vi "Load sxm File.vi"(8 "error in":errorcluster, 9 "Scan direction":bool=TRUE, 10 "Read channel":i8=-1 min=-1, 11 "Scan data file":path) -> (0 "error out":errorcluster, 1 "Data":sgl[][](array[numeric]) format="%#_5p", 2 "Channels info":T3, 3 "Scanfield":T2, 4 "Parameters":string[][](array[string]), 5 "Scan param":T1)   [LabVIEW 2017, in "Nanonis Prog Interface.lvlib"]
doc: "<B>Loads a Nanonis scan data (sxm) file.</B>\n\n<B>Scan data file</B>: path to the sxm file to load.\n<B>Read channel</B>: select which channel to read. If left unconnected, only the header information are read and no data are returned. To find out which channel to load you may run this function twice, using the <B>Channels config</B> output from the first run to determine the channel to load in the second run.\n<B>Scan direction</B>: defines whether to load the forward (True) or backward (False) data.\n\n\n<B>Scan param</B>: scan direction Up (True) or Down (False), scan speed in seconds per line, start time, and end time.\n<B>Channel data</B>: 2D-array containing the data of the specified channel and the given direction. The array element (0,0) corresponds to the top-left corner of the image.\n<B>Channels info</B>: list of channels available in the sxm file. Contains the channel name, calibration and offset. Use the channel indice in the <B>Read channel</B> input to load the data of that channel. Using calibration and offset you can calculate the voltage from the physical data.\n<B>Scanfield</B>: dimension of the scan field (center X & center Y, angle, width & height) and scan resolution (pixels & lines).\n<B>Parameters</B>: rest of header information.\n\n- Nanonis Programming Interface -"
uses:
  Nanonis Prog Interface.lvlib
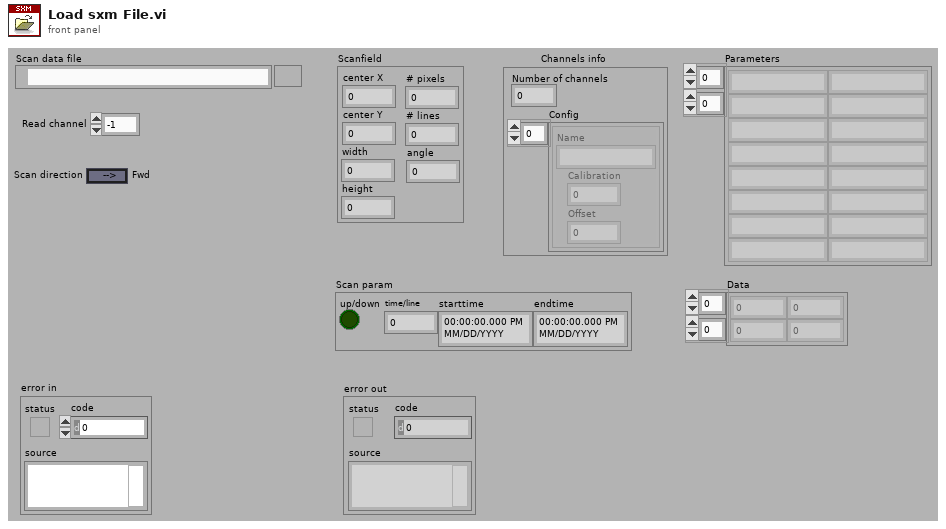
[diagram p1: front panel]
types:
  T1 = cluster{"up/down":bool, "time/line":sgl, "starttime":timestamp, "endtime":timestamp}
  T2 = cluster{"center X":sgl, "center Y":sgl, "angle":sgl, "width":sgl, "height":sgl, "# pixels":i32, "# lines":i32}
  T3 = cluster{"Number of channels":i8, "Config":cluster{"Name":string, "Calibration":sgl, "Offset":sgl}[]}
  T4 = enum16{"open", "replace", "create", "open or create", "replace or create", "replace or create with confirmation"}
  T5 = cluster{"Scanfield":cluster{"center X":sgl, "center Y":sgl, "width":sgl, "height":sgl, "angle":sgl}, "starttime":timestamp, "endtime":timestamp, "up/down":bool, "time/line":sgl, "selection":bool[], "# lines":i32, "# points":i32, "file":path, "channel config":cluster{"name":string, "calibration":sgl, "offset":sgl}[], "Parameters":string[][]}
  T6 = cluster{"name":string, "calibration":sgl, "offset":sgl}
  T7 = typedef "LVDateTimeRec.ctl" = cluster{"fractional second":dbl, "second":i32, "minute":i32, "hour":i32, "day of month":i32, "month":i32, "year":i32, "day of week":i32, "day of year":i32, "DST":i32}
  T8 = cluster{"name":string, "calibration":sgl, "offset":sgl}[]
  T9 = cluster{"center X":sgl, "center Y":sgl, "angle":sgl, "width":sgl, "height":sgl, "# points":i32, "# lines":i32}
  T10 = cluster{i32, "channel config":cluster{"name":string, "calibration":sgl, "offset":sgl}[]}
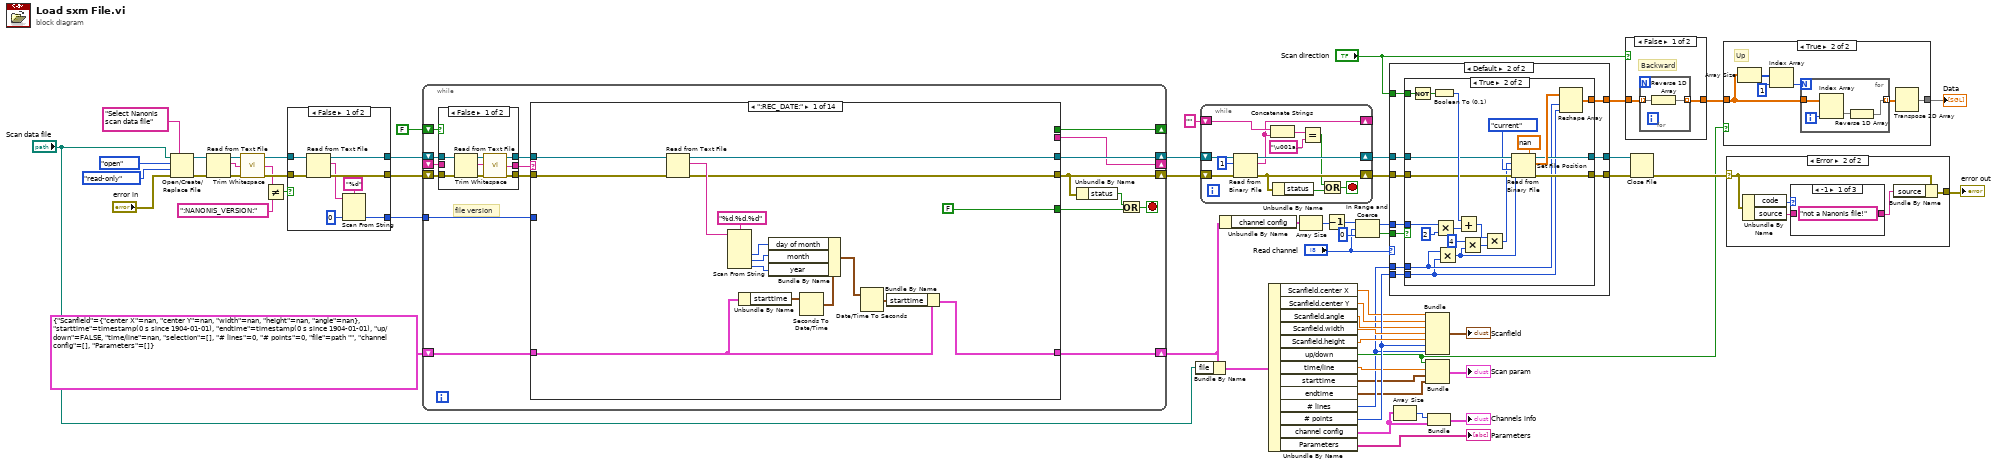
[diagram p0: block diagram]
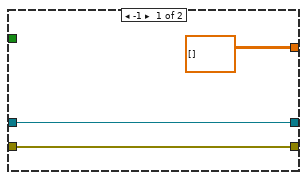
[diagram p4: hidden frame]
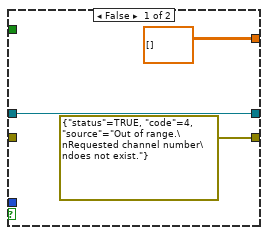
[diagram p5: hidden frame]
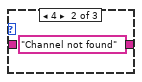
[diagram p7: hidden frame]
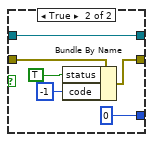
[diagram p9: hidden frame]
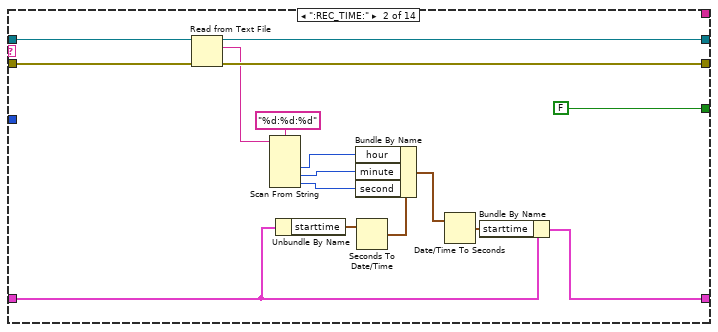
[diagram p11: hidden frame]
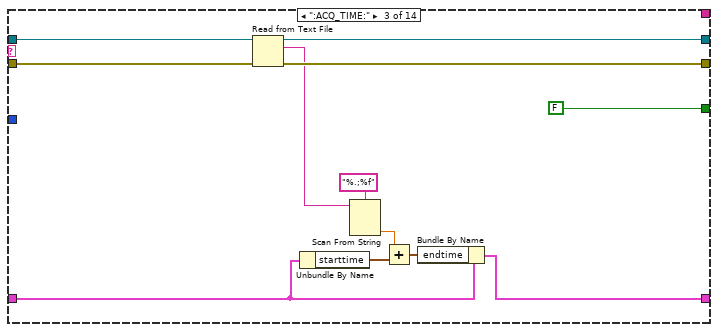
[diagram p12: hidden frame]
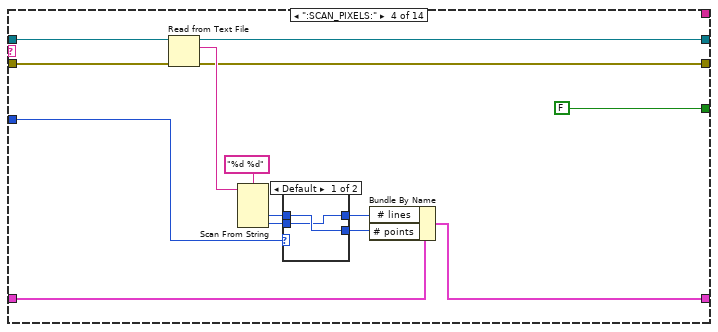
[diagram p13: hidden frame]
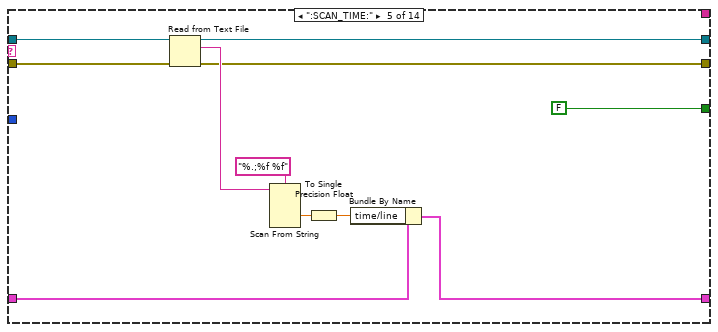
[diagram p15: hidden frame]
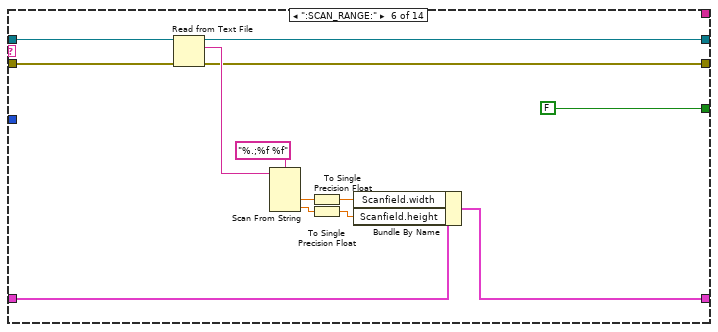
[diagram p16: hidden frame]
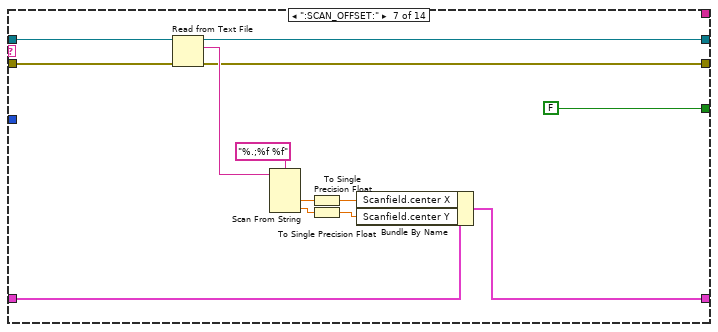
[diagram p17: hidden frame]
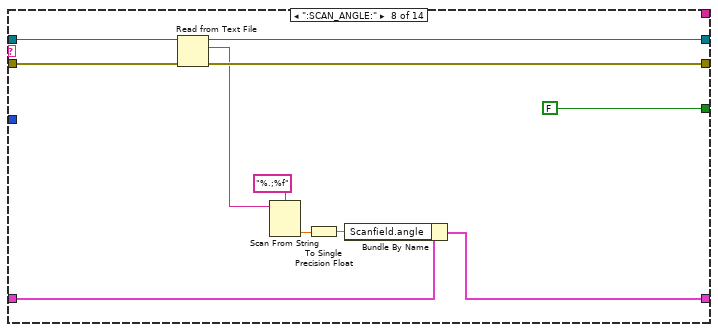
[diagram p18: hidden frame]
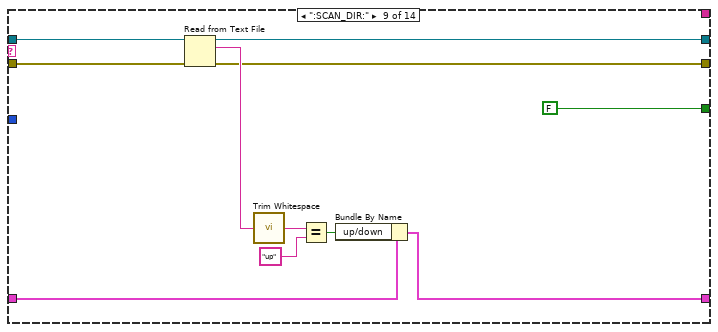
[diagram p19: hidden frame]
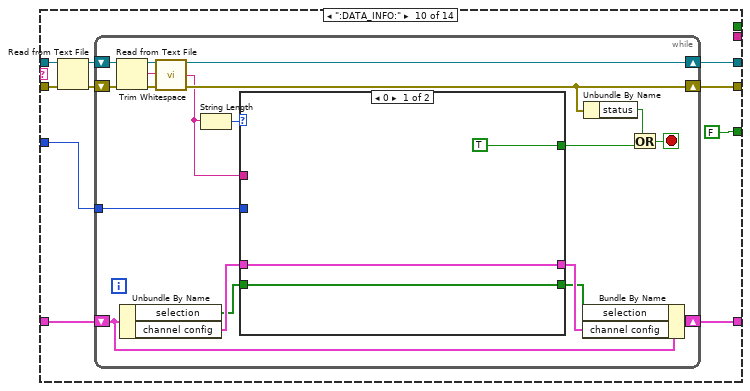
[diagram p20: hidden frame]
diagram:
  n1 = Open/Create/Replace File(file path (use dialog)="Scan data file", error in="error in", prompt="Select Nanonis scan data file", operation (0:open)=T4."open", access (0:read/write)=enum16{"read/write", "read-only", "write-only"}."read-only") -> (refnum out=w14:refnum<file>, error out=w15:errorcluster)  [unwired: 1 in, 1 out]
  n2 = Read from Text File(file (use dialog)=w14, error in=w15) -> (refnum out=w37:refnum<file>, text=w39:string, error out=w48:errorcluster)  [unwired: 2 in, 1 out]
  n3 = call <vilib>:"Trim Whitespace.vi"("string"=w39) -> ("trimmed string"=w38:string)  [unwired: 1 in]
  n4 = Not Equal?(x=w38, y=":NANONIS_VERSION:") -> (x != y?=w55:bool)
  n5 = case shown="False" w55 {
    tunnel: w48 -> [w58 w71]
    tunnel: [w65 w70] -> w47
    tunnel: w37 -> [w59 w68]
    tunnel: [w64 w68] -> w36
    tunnel: [w61 0 ("default value 1")] -> w35
    frame False {
      n6 = Read from Text File(file (use dialog)=w59, error in=w58) -> (refnum out=w64:refnum<file>, text=w62:string, error out=w65:errorcluster)  [unwired: 2 in, 1 out]
      n7 = Scan From String(format string="%d", input string=w62, default 1=0 ("default value 1")) -> (output 1=w61:i32)  [unwired: 2 in, 3 out]
    }
    frame True {
      n8 = Bundle By Name(cluster=w71, "status"=TRUE, "code"=-1) -> (w70:errorcluster)
    }
  }
  n9 = while {
    shift-right: [w87] -> w25
    shift-left: T5 {"Scanfield"={"center X"=nan, "center Y"=nan, "width"=nan, "height"=nan, "angle"=nan}, "starttime"=timestamp(0 s since 1904-01-01), "endtime"=timestamp(0 s since 1904-01-01), "up/down"=FALSE, "time/line"=nan, "selection"=[], "# lines"=0, "# points"=0, "file"=path "", "channel config"=[], "Parameters"=[]} ("Scan-Databuffer-attributes") -> [w88]
    shift-right: [w83] -> w52
    shift-left: w47 -> [w76]
    shift-right: [w79] -> w54
    shift-left: w36 -> [w77]
    tunnel: w35 -> [w78]
    shift-right: [w73] -> _
    shift-left: FALSE -> [w75]
    shift-right: [w72] -> _
    shift-left: _ -> [w74]
    stop <- w84 stop-if-true
    # "file version"
    n10 = case shown="False" w75 {
      tunnel: [w93 w96] -> w82
      tunnel: [w92 w95] -> w81
      tunnel: [w91 w97] -> w80
      tunnel: w77 -> [w90 w95]
      tunnel: w76 -> [w89 w96]
      tunnel: w74 -> [_ w97]
      frame False {
        n11 = Read from Text File(file (use dialog)=w90, error in=w89) -> (refnum out=w92:refnum<file>, text=w94:string, error out=w93:errorcluster)  [unwired: 2 in, 1 out]
        n12 = call <vilib>:"Trim Whitespace.vi"("string"=w94) -> ("trimmed string"=w91:string)  [unwired: 1 in]
      }
      frame True {
      }
    }
    n13 = case shown="\":REC_DATE:\"" w80 {
      selector: w80 -> [_ _ _ _ _ _ _ _ _ _ _ _ _ w347]
      tunnel: w81 -> [w101 w116 w131 w143 w161 w172 w185 w197 w209 w220 w311 w332 w344 w371]
      tunnel: [FALSE ("true") FALSE ("true") FALSE ("true") FALSE ("true") FALSE ("true") FALSE ("true") FALSE ("true") FALSE ("true") FALSE ("true") FALSE ("true") FALSE ("true") FALSE ("true") TRUE ("true") FALSE ("true")] -> w85
      tunnel: w88 -> [w112 w128 w141 w155 w170 w183 w196 w207 w218 w223 w303 w316 w345 w367]
      tunnel: [w111 w127 w140 w154 w169 w182 w195 w206 w217 w222 w301 w315 w345 w365] -> w87
      tunnel: [w104 w120 w133 w151 w165 w177 w190 w202 w212 w228 w313 w334 w344 w364] -> w79
      tunnel: w82 -> [w100 w117 w130 w142 w160 w171 w184 w198 w208 w219 w310 w331 w343 w370]
      tunnel: [w102 w119 w134 w149 w163 w175 w188 w201 w210 w224 w312 w333 w343 w363] -> w83
      tunnel: w78 -> [_ _ _ w144 _ _ _ _ _ w221 _ _ _ _]
      tunnel: [_ _ _ _ _ _ _ _ _ _ _ _ _ w362] -> w72
      tunnel: [_ _ _ _ _ _ _ _ _ _ _ _ _ w361] -> w73
      frame ":REC_DATE:" {
        n14 = Read from Text File(file (use dialog)=w101, error in=w100) -> (refnum out=w104:refnum<file>, text=w103:string, error out=w102:errorcluster)  [unwired: 2 in, 1 out]
        n15 = Scan From String(format string="%d.%d.%d", input string=w103) -> (output 1=w108:i32, output 2=w107:i32, output 3=w106:i32)  [unwired: 5 in, 3 out]
        n16 = Unbundle By Name(w112) -> ("starttime"=w99:timestamp)
        n17 = Seconds To Date/Time(time stamp (now)=w99) -> (date time rec=w113:T7)  [unwired: 1 in]
        n18 = Bundle By Name(cluster=w113, "day of month"=w108, "month"=w107, "year"=w106) -> (w98:T7)
        n19 = Date/Time To Seconds(2:w98) -> (0:w110:timestamp)  [unwired: 1 in]
        n20 = Bundle By Name(cluster=w112, "starttime"=w110) -> (w111:T5)
      }
      frame ":REC_TIME:" {
        n21 = Read from Text File(file (use dialog)=w116, error in=w117) -> (refnum out=w120:refnum<file>, text=w118:string, error out=w119:errorcluster)  [unwired: 2 in, 1 out]
        n22 = Scan From String(format string="%d:%d:%d", input string=w118) -> (output 1=w124:i32, output 2=w123:i32, output 3=w122:i32)  [unwired: 5 in, 3 out]
        n23 = Unbundle By Name(w128) -> ("starttime"=w115:timestamp)
        n24 = Seconds To Date/Time(time stamp (now)=w115) -> (date time rec=w129:T7)  [unwired: 1 in]
        n25 = Bundle By Name(cluster=w129, "hour"=w124, "minute"=w123, "second"=w122) -> (w114:T7)
        n26 = Date/Time To Seconds(2:w114) -> (0:w126:timestamp)  [unwired: 1 in]
        n27 = Bundle By Name(cluster=w128, "starttime"=w126) -> (w127:T5)
      }
      frame ":ACQ_TIME:" {
        n28 = Read from Text File(file (use dialog)=w131, error in=w130) -> (refnum out=w133:refnum<file>, text=w132:string, error out=w134:errorcluster)  [unwired: 2 in, 1 out]
        n29 = Unbundle By Name(w141) -> ("starttime"=w137:timestamp)
        n30 = Scan From String(format string="%.;%f", input string=w132) -> (output 1=w135:dbl)  [unwired: 3 in, 3 out]
        n31 = Add(x=w135, y=w137) -> (x+y=w136:timestamp)
        n32 = Bundle By Name(cluster=w141, "endtime"=w136) -> (w140:T5)
      }
      frame ":SCAN_PIXELS:" {
        n33 = Read from Text File(file (use dialog)=w143, error in=w142) -> (refnum out=w151:refnum<file>, text=w150:string, error out=w149:errorcluster)  [unwired: 2 in, 1 out]
        n34 = Scan From String(format string="%d %d", input string=w150) -> (output 1=w148:i32, output 2=w147:i32)  [unwired: 4 in, 3 out]
        n35 = case shown="Default" w144 {
          tunnel: w148 -> [w157 w159]
          tunnel: w147 -> [w156 w158]
          tunnel: [w156 w159] -> w146
          tunnel: [w157 w158] -> w145
          frame Default {
          }
          frame 0, 1 {
          }
        }
        n36 = Bundle By Name(cluster=w155, "# lines"=w146, "# points"=w145) -> (w154:T5)
      }
      frame ":SCAN_TIME:" {
        n37 = Read from Text File(file (use dialog)=w161, error in=w160) -> (refnum out=w165:refnum<file>, text=w164:string, error out=w163:errorcluster)  [unwired: 2 in, 1 out]
        n38 = Scan From String(format string="%.;%f %f", input string=w164) -> (output 1=w167:dbl)  [unwired: 5 in, 3 out]
        n39 = To Single Precision Float(number=w167) -> (single precision float=w162:sgl)
        n40 = Bundle By Name(cluster=w170, "time/line"=w162) -> (w169:T5)
      }
      frame ":SCAN_RANGE:" {
        n41 = Read from Text File(file (use dialog)=w172, error in=w171) -> (refnum out=w177:refnum<file>, text=w176:string, error out=w175:errorcluster)  [unwired: 2 in, 1 out]
        n42 = Scan From String(format string="%.;%f %f", input string=w176) -> (output 1=w180:dbl, output 2=w179:dbl)  [unwired: 4 in, 3 out]
        n43 = To Single Precision Float(number=w180) -> (single precision float=w174:sgl)
        n44 = To Single Precision Float(number=w179) -> (single precision float=w173:sgl)
        n45 = Bundle By Name(cluster=w183, "Scanfield.width"=w174, "Scanfield.height"=w173) -> (w182:T5)
      }
      frame ":SCAN_OFFSET:" {
        n46 = Read from Text File(file (use dialog)=w185, error in=w184) -> (refnum out=w190:refnum<file>, text=w189:string, error out=w188:errorcluster)  [unwired: 2 in, 1 out]
        n47 = Scan From String(format string="%.;%f %f", input string=w189) -> (output 1=w193:dbl, output 2=w192:dbl)  [unwired: 4 in, 3 out]
        n48 = To Single Precision Float(number=w193) -> (single precision float=w187:sgl)
        n49 = To Single Precision Float(number=w192) -> (single precision float=w186:sgl)
        n50 = Bundle By Name(cluster=w196, "Scanfield.center X"=w187, "Scanfield.center Y"=w186) -> (w195:T5)
      }
      frame ":SCAN_ANGLE:" {
        n51 = Read from Text File(file (use dialog)=w197, error in=w198) -> (refnum out=w202:refnum<file>, text=w200:string, error out=w201:errorcluster)  [unwired: 2 in, 1 out]
        n52 = Scan From String(format string="%.;%f", input string=w200) -> (output 1=w204:dbl)  [unwired: 3 in, 3 out]
        n53 = To Single Precision Float(number=w204) -> (single precision float=w199:sgl)
        n54 = Bundle By Name(cluster=w207, "Scanfield.angle"=w199) -> (w206:T5)
      }
      frame ":SCAN_DIR:" {
        n55 = Read from Text File(file (use dialog)=w209, error in=w208) -> (refnum out=w212:refnum<file>, text=w211:string, error out=w210:errorcluster)  [unwired: 2 in, 1 out]
        n56 = call <vilib>:"Trim Whitespace.vi"("string"=w211) -> ("trimmed string"=w215:string)  [unwired: 1 in]
        n57 = Equal?(x=w215, y="up") -> (x = y?=w213:bool)
        n58 = Bundle By Name(cluster=w218, "up/down"=w213) -> (w217:T5)
      }
      frame ":DATA_INFO:" {
        n59 = Read from Text File(file (use dialog)=w220, error in=w219) -> (refnum out=w226:refnum<file>, error out=w225:errorcluster)  [unwired: 2 in, 2 out]
        n60 = while {
          shift-right: [w235] -> w222
          shift-left: w223 -> [w236]
          shift-right: [w242] -> w224
          shift-left: w225 -> [w229]
          shift-right: [w244] -> w228
          shift-left: w226 -> [w230]
          tunnel: w221 -> [w231]
          stop <- w239 stop-if-true
          n61 = Read from Text File(file (use dialog)=w230, error in=w229) -> (refnum out=w244:refnum<file>, text=w243:string, error out=w242:errorcluster)  [unwired: 2 in, 1 out]
          n62 = Unbundle By Name(w236) -> ("selection"=w234:bool[], "channel config"=w238:T8)
          n63 = call <vilib>:"Trim Whitespace.vi"("string"=w243) -> ("trimmed string"=w232:string)  [unwired: 1 in]
          n64 = String Length(string=w232) -> (length=w245:i32)
          n65 = case shown="0" w245 {
            tunnel: w238 -> [w248 w255]
            tunnel: [w248 w254] -> w237
            tunnel: [TRUE w253] -> w240
            tunnel: w234 -> [w246 w252]
            tunnel: [w246 w251] -> w233
            tunnel: w232 -> [_ w250]
            tunnel: w231 -> [_ w249]
            frame 0 {
            }
            frame Default {
              n66 = case shown="Default" w249 {
                tunnel: w255 -> [w274 w294]
                tunnel: [w272 w292] -> w254
                tunnel: [FALSE FALSE] -> w253
                tunnel: w252 -> [w268 w288]
                tunnel: [w266 w286] -> w251
                tunnel: w250 -> [w256 w277]
                frame 0, 1 {
                  w262 = "%.; %d%s%s%s%e%e"  # Read strings (no whitespace allowed)
                  n67 = Scan From String(format string=w262, input string=w256) -> (output 1=w261:i32, output 2=w260:string, output 3=w259:string, output 5=w258:dbl, output 6=w257:dbl)  [unwired: 9 in, 3 out]
                  n68 = Replace Array Subset(array=w268, new element=TRUE ("new element/subarray"), index=w261) -> (w266:bool[])
                  n69 = Search and Replace String(replace all?=TRUE ("replace all? (F)"), input string=w260, search string="_", replace string=" " ("replace string (\"\")")) -> (result string=w264:string)  [unwired: 4 in, 3 out]
                  n70 = call <userlib>:"Append Unit to Signal Name.vi"("Unit"=w259, "Name"=w264) -> ("Name with unit"=w263:string)  [unwired: 5 in]
                  n71 = Bundle By Name(cluster=T6 {"name"="", "calibration"=0.0, "offset"=0.0} ("channel config"), "name"=w263, "calibration"=w258, "offset"=w257) -> (w273:T6)
                  n72 = Build Array (concatenate)(w274, w273) -> (w272:T8)
                }
                frame Default {
                  w276 = "%.;%d\t%[^\t]\t%[^\t]\t%s\t%e\t%e"  # Read tab-separated strings (spaces allowed)
                  n73 = Scan From String(format string=w276, input string=w277) -> (output 1=w282:i32, output 2=w281:string, output 3=w280:string, output 5=w279:dbl, output 6=w278:dbl)  [unwired: 9 in, 3 out]
                  n74 = Replace Array Subset(array=w288, new element=TRUE ("new element/subarray"), index=w282) -> (w286:bool[])
                  n75 = Search and Replace String(replace all?=TRUE ("replace all? (F)"), input string=w281, search string="_", replace string=" " ("replace string (\"\")")) -> (result string=w284:string)  [unwired: 4 in, 3 out]
                  n76 = call <userlib>:"Append Unit to Signal Name.vi"("Unit"=w280, "Name"=w284) -> ("Name with unit"=w283:string)  [unwired: 5 in]
                  n77 = Bundle By Name(cluster=T6 {"name"="", "calibration"=0.0, "offset"=0.0} ("channel config"), "name"=w283, "calibration"=w279, "offset"=w278) -> (w293:T6)
                  n78 = Build Array (concatenate)(w294, w293) -> (w292:T8)
                }
              }
            }
          }
          n79 = Bundle By Name(cluster=w236, "selection"=w233, "channel config"=w237) -> (w235:T5)
          n80 = Unbundle By Name(w242) -> ("status"=w241:bool)
          n81 = Or(x=w241, y=w240) -> (x .or. y?=w239:bool)
        }
      }
      frame ":BIAS:" {
        n82 = Read from Text File(file (use dialog)=w311, error in=w310) -> (refnum out=w313:refnum<file>, text=w297:string, error out=w312:errorcluster)  [unwired: 2 in, 1 out]
        n83 = call <vilib>:"Trim Whitespace.vi"("string"=w297) -> ("trimmed string"=w296:string)  [unwired: 1 in]
        n84 = Scan From String(format string="%.;%f", input string=w297) -> (error out=w300:errorcluster, output 1=w307:dbl)  [unwired: 3 in, 2 out]
        n85 = Format Value(format string="%#_6p", value (0)=w307) -> (output string=w299:string)  [unwired: 1 in]
        n86 = Unbundle By Name(w303) -> ("Parameters"=w309:string[][])
        n87 = Select(t=w296, s=w300, f=w299) -> (s? t:f=w298:string)
        n88 = Build Array("Bias (V)" ("element"), w298) -> (w304:string[])
        n89 = Build Array (concatenate)(w309, w304) -> (w302:string[][])
        n90 = Bundle By Name(cluster=w303, "Parameters"=w302) -> (w301:T5)
      }
      frame ":Z-CONTROLLER:" {
        w322 = string[] []
        w323 = "%s" ("format string")
        w324 = "\t"
        n91 = Read from Text File(file (use dialog)=w332, error in=w331) -> (refnum out=w330:refnum<file>, text=w328:string, error out=w329:errorcluster)  [unwired: 2 in, 1 out]
        n92 = call <vilib>:"Trim Whitespace.vi"("string"=w328) -> ("trimmed string"=w326:string)  [unwired: 1 in]
        n93 = Spreadsheet String To Array(delimiter (Tab)=w324, format string=w323, spreadsheet string=w326, array type (2D Dbl)=w322) -> (array=w320:string[])
        n94 = Read from Text File(file (use dialog)=w330, error in=w329) -> (refnum out=w334:refnum<file>, text=w327:string, error out=w333:errorcluster)  [unwired: 2 in, 1 out]
        n95 = call <vilib>:"Trim Whitespace.vi"("string"=w327) -> ("trimmed string"=w325:string)  [unwired: 1 in]
        n96 = Spreadsheet String To Array(delimiter (Tab)=w324, format string=w323, spreadsheet string=w325, array type (2D Dbl)=w322) -> (array=w319:string[])
        n97 = Unbundle By Name(w316) -> ("Parameters"=w318:string[][])
        n98 = for {
          tunnel: "Z-Ctrl: " ("string") -> [w342]
          tunnel: w320 -> [w341] mode=indexing
          tunnel: w319 -> [w339] mode=indexing
          shift-right: [w338] -> w317
          shift-left: w318 -> [w337]
          n99 = Concatenate Strings(w342, w341) -> (w340:string)
          n100 = Build Array(w340, w339) -> (w336:string[])
          n101 = Build Array (concatenate)(w337, w336) -> (w338:string[][])
        }
        n102 = Bundle By Name(cluster=w316, "Parameters"=w317) -> (w315:T5)
      }
      frame ":SCANIT_END:" {
      }
      frame Default {
        n103 = while {
          tunnel: w371 -> [w385]
          tunnel: w370 -> [w384]
          tunnel: [w383] -> w364
          tunnel: [w380] -> w363
          tunnel: [w373] -> w362
          tunnel: [w377] -> w361
          shift-right: [w374] -> w359
          shift-left: "" -> [w375]
          stop <- w379 stop-if-true
          n104 = Read from Text File(file (use dialog)=w385, error in=w384) -> (refnum out=w383:refnum<file>, text=w376:string, error out=w380:errorcluster)  [unwired: 2 in, 1 out]
          n105 = Match Pattern(string=w376, regular expression="^:.*:") -> (match substring=w373:string, offset past match=w381:i32)  [unwired: 1 in, 2 out]
          n106 = Unbundle By Name(w380) -> ("status"=w378:bool)
          n107 = Greater Or Equal To 0?(x=w381) -> (x >= 0?=w377:bool)
          n108 = Or(x=w377, y=w378) -> (x .or. y?=w379:bool)
          n109 = case shown="False" w377 {
            tunnel: w376 -> [w388 _]
            tunnel: w375 -> [w387 w389]
            tunnel: [w386 w389] -> w374
            frame False {
              n110 = Concatenate Strings(w387, w388) -> (w386:string)
            }
            frame True {
            }
          }
        }
        n111 = String Length(string=w347) -> (length=w353:i32)
        n112 = Subtract(x=w353, y=2) -> (x-y=w351:i32)
        n113 = String Subset(string=w347, offset (0)=1, length (rest)=w351) -> (substring=w350:string)
        n114 = Match Pattern(string=w347, regular expression=":.*:") -> (offset past match=w356:i32)  [unwired: 1 in, 3 out]
        n115 = Empty String/Path?(string/path=w347) -> (empty?=w369:bool)
        n116 = Less Than 0?(x=w356) -> (x < 0?=w355:bool)
        n117 = Unbundle By Name(w367) -> ("Parameters"=w368:string[][])
        n118 = call <vilib>:"Trim Whitespace.vi"("string"=w359) -> ("trimmed string"=w349:string)  [unwired: 1 in]
        n119 = Select(t=w347, s=w355, f=w350) -> (s? t:f=w348:string)
        n120 = Build Array(w348, w349) -> (w358:string[])
        n121 = case shown="False" w369 {
          tunnel: w368 -> [w391 w393]
          tunnel: [w392 w393] -> w366
          tunnel: w358 -> [w390 _]
          frame False {
            n122 = Build Array (concatenate)(w391, w390) -> (w392:string[][])
          }
          frame True {
          }
        }
        n123 = Bundle By Name(cluster=w367, "Parameters"=w366) -> (w365:T5)
      }
    }
    n124 = Unbundle By Name(w83) -> ("status"=w86:bool)
    n125 = Or(x=w86, y=w85) -> (x .or. y?=w84:bool)
  }
  n126 = Bundle By Name(cluster=w25, "file"="Scan data file") -> (w34:T5)
  n127 = while {
    shift-right: [w400] -> _
    shift-left: "" -> [w405]
    shift-right: [w401] -> w50
    shift-left: w52 -> [w395]
    shift-right: [w403] -> w51
    shift-left: w54 -> [w396]
    stop <- w397 stop-if-true
    n128 = Read from Binary File(8:w395, 10:1 ("count"), 11:w396) -> (0:w401:errorcluster, 2:w400:string, 3:w403:refnum<file>)  [unwired: 3 in, 1 out]
    n129 = Concatenate Strings(w405, w400) -> (w404:string)
    n130 = Unbundle By Name(w401) -> ("status"=w399:bool)
    n131 = Equal?(x=w404, y="\u001a\u0004") -> (x = y?=w398:bool)
    n132 = Or(x=w398, y=w399) -> (x .or. y?=w397:bool)
  }
  n133 = Unbundle By Name(w25) -> ("channel config"=w44:T8)
  n134 = Unbundle By Name(w34) -> ("Scanfield.center X"=w12:sgl, "Scanfield.center Y"=w11:sgl, "Scanfield.angle"=w10:sgl, "Scanfield.width"=w30:sgl, "Scanfield.height"=w29:sgl, "up/down"=w21:bool, "time/line"=w27:sgl, "starttime"=w3:timestamp, "endtime"=w2:timestamp, "# lines"=w4:i32, "# points"=w28:i32, "channel config"=w13:T8, "Parameters"=→"Parameters":string[][])
  n135 = Array Size(array=w44) -> (size(s)=w43:i32)
  n136 = Decrement(x=w43) -> (x-1=w42:i32)
  n137 = In Range and Coerce(upper limit=w42, x="Read channel", lower limit=0) -> (coerced(x)=w41:i32, In Range?=w26:bool)
  n138 = case shown="Default" "Read channel" {
    tunnel: "Scan direction" -> [_ w418]
    tunnel: w51 -> [w407 w417]
    tunnel: w50 -> [w406 w416]
    tunnel: [w407 w415] -> w49
    tunnel: [sgl[][] [] w414] -> w46
    tunnel: w41 -> [_ w413]
    tunnel: [w406 w412] -> w33
    tunnel: w4 -> [_ w411]
    tunnel: w28 -> [_ w410]
    tunnel: w26 -> [_ w409]
    frame -1 {
    }
    frame Default {
      n139 = case shown="True" w409 {
        tunnel: w418 -> [_ w441]
        tunnel: w417 -> [w420 w440]
        tunnel: w416 -> [_ w439]
        tunnel: [w420 w437] -> w415
        tunnel: [sgl[][] [] w436] -> w414
        tunnel: w413 -> [_ w435]
        tunnel: [errorcluster {"status"=TRUE, "code"=4, "source"="Out of range.\nRequested channel number\ndoes not exist."} ("error out") w427] -> w412
        tunnel: w411 -> [_ w426]
        tunnel: w410 -> [_ w425]
        frame False {
        }
        frame True {
          n140 = Not(x=w441) -> (.not. x?=w422:bool)
          n141 = Boolean To (0,1)(Boolean=w422) -> (0, 1=w444:i16)
          n142 = Multiply(x=w435, y=2) -> (x*y=w443:i32)
          n143 = Multiply(x=w426, y=w425) -> (x*y=w430:i32)
          n144 = Add(x=w444, y=w443) -> (x+y=w429:i32)
          n145 = Multiply(x=4 ("y"), y=w430) -> (x*y=w432:i32)
          n146 = Multiply(x=w429, y=w432) -> (x*y=w428:i32)
          n147 = Set File Position(offset (in bytes) (0)=w428, refnum=w440, from (0:start)=enum16{"start", "end", "current"}."current" ("pos mode (0:2)"), error in=w439) -> (refnum out=w424:refnum<file>, error out=w423:errorcluster)
          n148 = Read from Binary File(5:sgl nan ("element"), 8:w423, 10:w430, 11:w424) -> (0:w427:errorcluster, 2:w438:sgl[], 3:w437:refnum<file>)  [unwired: 2 in, 1 out]
          n149 = Reshape Array(w438, w426, w425) -> (w436:sgl[][])
        }
      }
    }
  }
  n150 = Array Size(array=w13) -> (size(s)=w24:i32)
  n151 = Bundle("center X"=w12, "center Y"=w11, "angle"=w10, "width"=w30, "height"=w29, "# points"=w28, "# lines"=w4) -> (→"Scanfield":T9)  [unwired: 1 in]
  n152 = Bundle("up/down"=w21, "time/line"=w27, "starttime"=w3, "endtime"=w2) -> (→"Scan param":T1)  [unwired: 1 in]
  n153 = Bundle(w24, "channel config"=w13) -> (→"Channels info":T10)  [unwired: 1 in]
  n154 = case shown="False" "Scan direction" {
    tunnel: w46 -> [w446 w449]
    tunnel: [w445 w449] -> w20
    frame False {
      # "Backward"
      n155 = for {
        tunnel: w446 -> [w448] mode=indexing
        tunnel: [w447] -> w445 mode=indexing
        n156 = Reverse 1D Array(array=w448) -> (reversed array=w447:sgl[])
      }
    }
    frame True {
      # "Forward"
    }
  }
  n157 = Close File(refnum=w49, error in=w33) -> (error out=w45:errorcluster)  [unwired: 1 out]
  n158 = case shown="True" w21 {
    tunnel: w20 -> [w450 w453]
    tunnel: [w450 w451] -> w19
    frame False {
      # "Down"
    }
    frame True {
      # "Up"
      n159 = Array Size(array=w453) -> (size(s)=w456:i32[])
      n160 = Index Array(array=w456, index=1) -> (element=w454:i32)
      n161 = for {
        N: w454 -> [_]
        tunnel: w453 -> [w460]
        tunnel: [w457] -> w452 mode=indexing
        i -> [w459]
        n162 = Index Array(array=w460, index (col)=w459) -> (element=w458:sgl[])  [unwired: 1 in]
        n163 = Reverse 1D Array(array=w458) -> (reversed array=w457:sgl[])
      }
      n164 = Transpose 2D Array(2D array=w452) -> (transposed array=w451:sgl[][])
    }
  }
  "Data" <- w19
  n165 = case shown="Error" w45 {
    selector: w45 -> [w461 w462]
    tunnel: [w461 w465] -> w32
    frame No Error {
    }
    frame Error {
      n166 = Unbundle By Name(w462) -> ("code"=w464:i32, "source"=w463:string)
      n167 = case shown="-1" w464 {
        tunnel: ["not a Nanonis file!" ("message") "Channel not found" ("message") w469] -> w466
        tunnel: w463 -> [_ _ w469]
        frame -1 {
        }
        frame 4 {
        }
        frame Default {
        }
      }
      n168 = Bundle By Name(cluster=w462, "source"=w466) -> (w465:errorcluster)
    }
  }
  "error out" <- w32
